vi "Double FFT Mesurament (Max Bin detection - Control - Init Wave&Window - Snapshot - DoubleFFT - Latency) test.vi"() -> ()   [LabVIEW 2014]
uses:
  <vilib>/Platform/TimedLoop/XDataNode/timing_clust.ctl
  <vilib>/Platform/TimedLoop/XDataNode/nitl_modes.ctl
  <vilib>/Platform/TimedLoop/XDataNode/wakeup.ctl
  <vilib>/rvi/Analysis/measure/FFT/simModelSupport/niFPGA FFT Streaming Sim Properties.ctl
  <vilib>/rvi/Analysis/measure/FFT/simModelSupport/niFPGA FFT Sim Stream Group Properties.ctl
  <vilib>/rvi/Analysis/measure/FFT/simModelSupport/niFPGA FFT Sim Types.ctl
  <vilib>/rvi/Analysis/measure/FFT/simModelSupport/niFpgaFFTSimArithmeticProperties.ctl
  <vilib>/rvi/Analysis/measure/FFT/simModelSupport/niFpgaFFTSimDfxp.ctl
  <vilib>/fxp/LVFixedPointQuantizationPolicyTypeDef.ctl
  <vilib>/rvi/Analysis/measure/FFT/XNode/niFpgaFFTButterflyDelays.ctl
  <vilib>/rvi/Emulation/niFpgaSctlEmulationGetInTimedLoop.vi
  <vilib>/rvi/Emulation/niFpgaEmulationReportErrorSimple.vi
  <vilib>/rvi/Emulation/niFpgaGetClockAttributes.vi
  <vilib>/rvi/Emulation/niFpgaCriticalErrorInLSC.vi
  <vilib>/rvi/Emulation/niFpgaEmulationIsFPGAContextNoSignature.vi
  <vilib>/rvi/DataTransferAndStorage/Container/Common/niFpgaContainerGetUniqueNameForEmu.vi
  <vilib>/rvi/Memory/Memory_Emulation/niFpgaMemoryEmulationCacheClearOnFirstRun.vi
  <vilib>/rvi/Memory/Memory_Emulation/nirvimemoryEmulationManagerCache_MakeExclusive.vi
  <vilib>/rvi/Memory/Memory_Emulation/niFpgaMemoryEmulationValidateCache.vi
  <vilib>/rvi/Memory/Memory_Emulation/nirvimemoryEmulationManagerCache_InsertValue.vi
  <vilib>/Utility/error.llb/Clear Errors.vi
  <vilib>/rvi/Memory/Memory_Emulation/nirvimemoryEmulationManagerCache_ReleaseExclusive.vi
  <vilib>/rvi/Memory/Memory_Emulation/nirvimemoryEmulationManagerCache_GetValue.vi
  <vilib>/rvi/Memory/Memory_Emulation/nirvimemoryEmulationManagerCache_SetValue.vi
  <vilib>/rvi/Emulation/niFpgaProcessEmulError.vi
  <vilib>/rvi/errors/niFpgaSetErrorForExecOnDevCompSimple.vi
  <vilib>/rvi/eio/common/nirviEmuReportErrorAndStop.vi
  <vilib>/rvi/FIFO/Fifo_Resource/nirvififoEmulationSetSize.vi
  <vilib>/rvi/FIFO/Fifo_Resource/nirviFifoEmulationQueueMgr.vi
  <instcachedir>/0/nirviFifoEmulationQueueMgr_E5CAEC123FF24DC58D834DCA3CDAA9B5.lvgen/nirviFifoEmulationQueueMgr_E5CAEC123FF24DC58D834DCA3CDAA9B5_012.vi
  <vilib>/rvi/FIFO/Fifo_Resource/nirvififoEmulationCreateLock.vi
  <vilib>/rvi/FIFO/Fifo_Resource/nirvififoEmulationObtainLock.vi
  <vilib>/rvi/FIFO/Fifo_Resource/nirvififoEmulationReleaseLock.vi
  <vilib>/rvi/occurrence/nirviWaitOnOccurrenceBase.vi
  <vilib>/rvi/errors/nirviReportUnexpectedCaseInternalError.vi
  <vilib>/rvi/errors/nirviReportUnexpectedCaseInternalError (U32).vi
  <instcachedir>/0/nirviFifoEmulationQueueMgr_E5CAEC123FF24DC58D834DCA3CDAA9B5.lvgen/nirviFifoEmulationQueueMgr_E5CAEC123FF24DC58D834DCA3CDAA9B5_010.vi
  <vilib>/rvi/FIFO/Fifo_Resource/nirvififoEmulationDetermineInputValidOut.vi
  <vilib>/rvi/Memory/Memory_Emulation/nirvimemoryFastEmulation.vi
  <vilib>/rvi/Memory/Memory_Emulation/nirvimemoryEmulation.vi
  <vilib>/rvi/Analysis/measure/FFT/simModelSupport/niFpgaFFTSimModelStreamingCore.vi
  <vilib>/rvi/interface/RandomDataEmulation/niFpgaRandomDataHandleErrors.vi
  <vilib>/rvi/eio/common/nirviEmuTemplateMethod_errors.vi
  <vilib>/Platform/TimedLoop/XDataNode/XDataNode.xnode
  <vilib>/rvi/DataTransferAndStorage/Container/XNode/niFpgaContainer.xnode
  <vilib>/rvi/DataTransferAndStorage/Register/Emulation/niFpgaRegisterEmulation.vi
  <vilib>/rvi/FIFO/Fifo_Resource/nirvififoEmulationRead.vi
  <vilib>/rvi/FIFO/Fifo_Resource/nirvififoEmulationWrite.vi
  <vilib>/rvi/FIFO/Fifo_Resource/nirvififoEmulationGetNumberOfElementsToWrite.vi
  <vilib>/rvi/Analysis/measure/FFT/XNode/niFpgaFFT.xnode
  <vilib>/rvi/interface/RandomDataEmulation/nirviRandomDataFpgaReadWriteTemplate.vi
  <vilib>/eio/EIOMethodNode/EIOMethodNode.xnode
  <vilib>/Platform/TimedLoop/XDataNode/XDNodeRunTimeDep.lvlib
panel:
  in  "Latency points":u32
  in  "snapshot":bool
  in  "first bin":i32=4
  in  "last bin":i32=251
  in  "lower limit 2":u32=682
  in  "lower limit 1":u32=57
  in  "upper limit 2":u32=1193
  in  "upper limit 1":u32=568
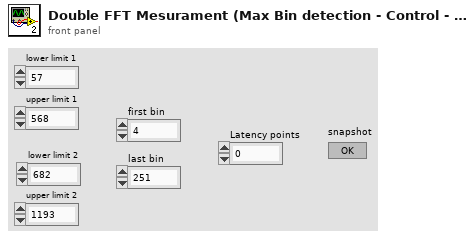
[diagram p1: front panel]
types:
  T1 = typedef "XDNodeRunTimeDep.lvlib/timing_clust.ctl" = cluster{"Expected End [f-1]":u64, "Actual End [f-1]":u64, "Finished Late? [f-1]":bool, "Expected End [i-1]":u64, "Actual End [i-1]":u64, "Finished Late? [i-1]":bool, "Expected Start [i]":u64, "Actual Start [i]":u64, "Expected Start [f]":u64, "Actual Start [f]":u64, "Source Name":string, "Structure Name":string, "Period":i64, "Deadline":i64, "Offset":i64, "Start":i64, "Priority":i32, "Timeout":i32, "Mode":T2, "Wakeup Reason":T3, "Error":errorcluster, "Source Type":string, "Secondary Source Type":string, "Global End Time":u64, "Global Start Time":u64, "Frame Duration":u64, "Iteration Duration":u64, "Assigned CPU":i32, "I/O Scan Engine Mode":u32}
  T2 = typedef "XDNodeRunTimeDep.lvlib/nitl_modes.ctl" = enum32{"No Change", "Process missed periods, maintain original phase", "Discard missed periods, maintain original phase", "Process missed periods, ignore original phase", "Discard missed periods, ignore original phase"}
  T3 = typedef "XDNodeRunTimeDep.lvlib/wakeup.ctl" = enum32{"Normal", "Aborted", "Asynchronous wakeup", "Timing source error", "Timed loop error", "Timeout"}
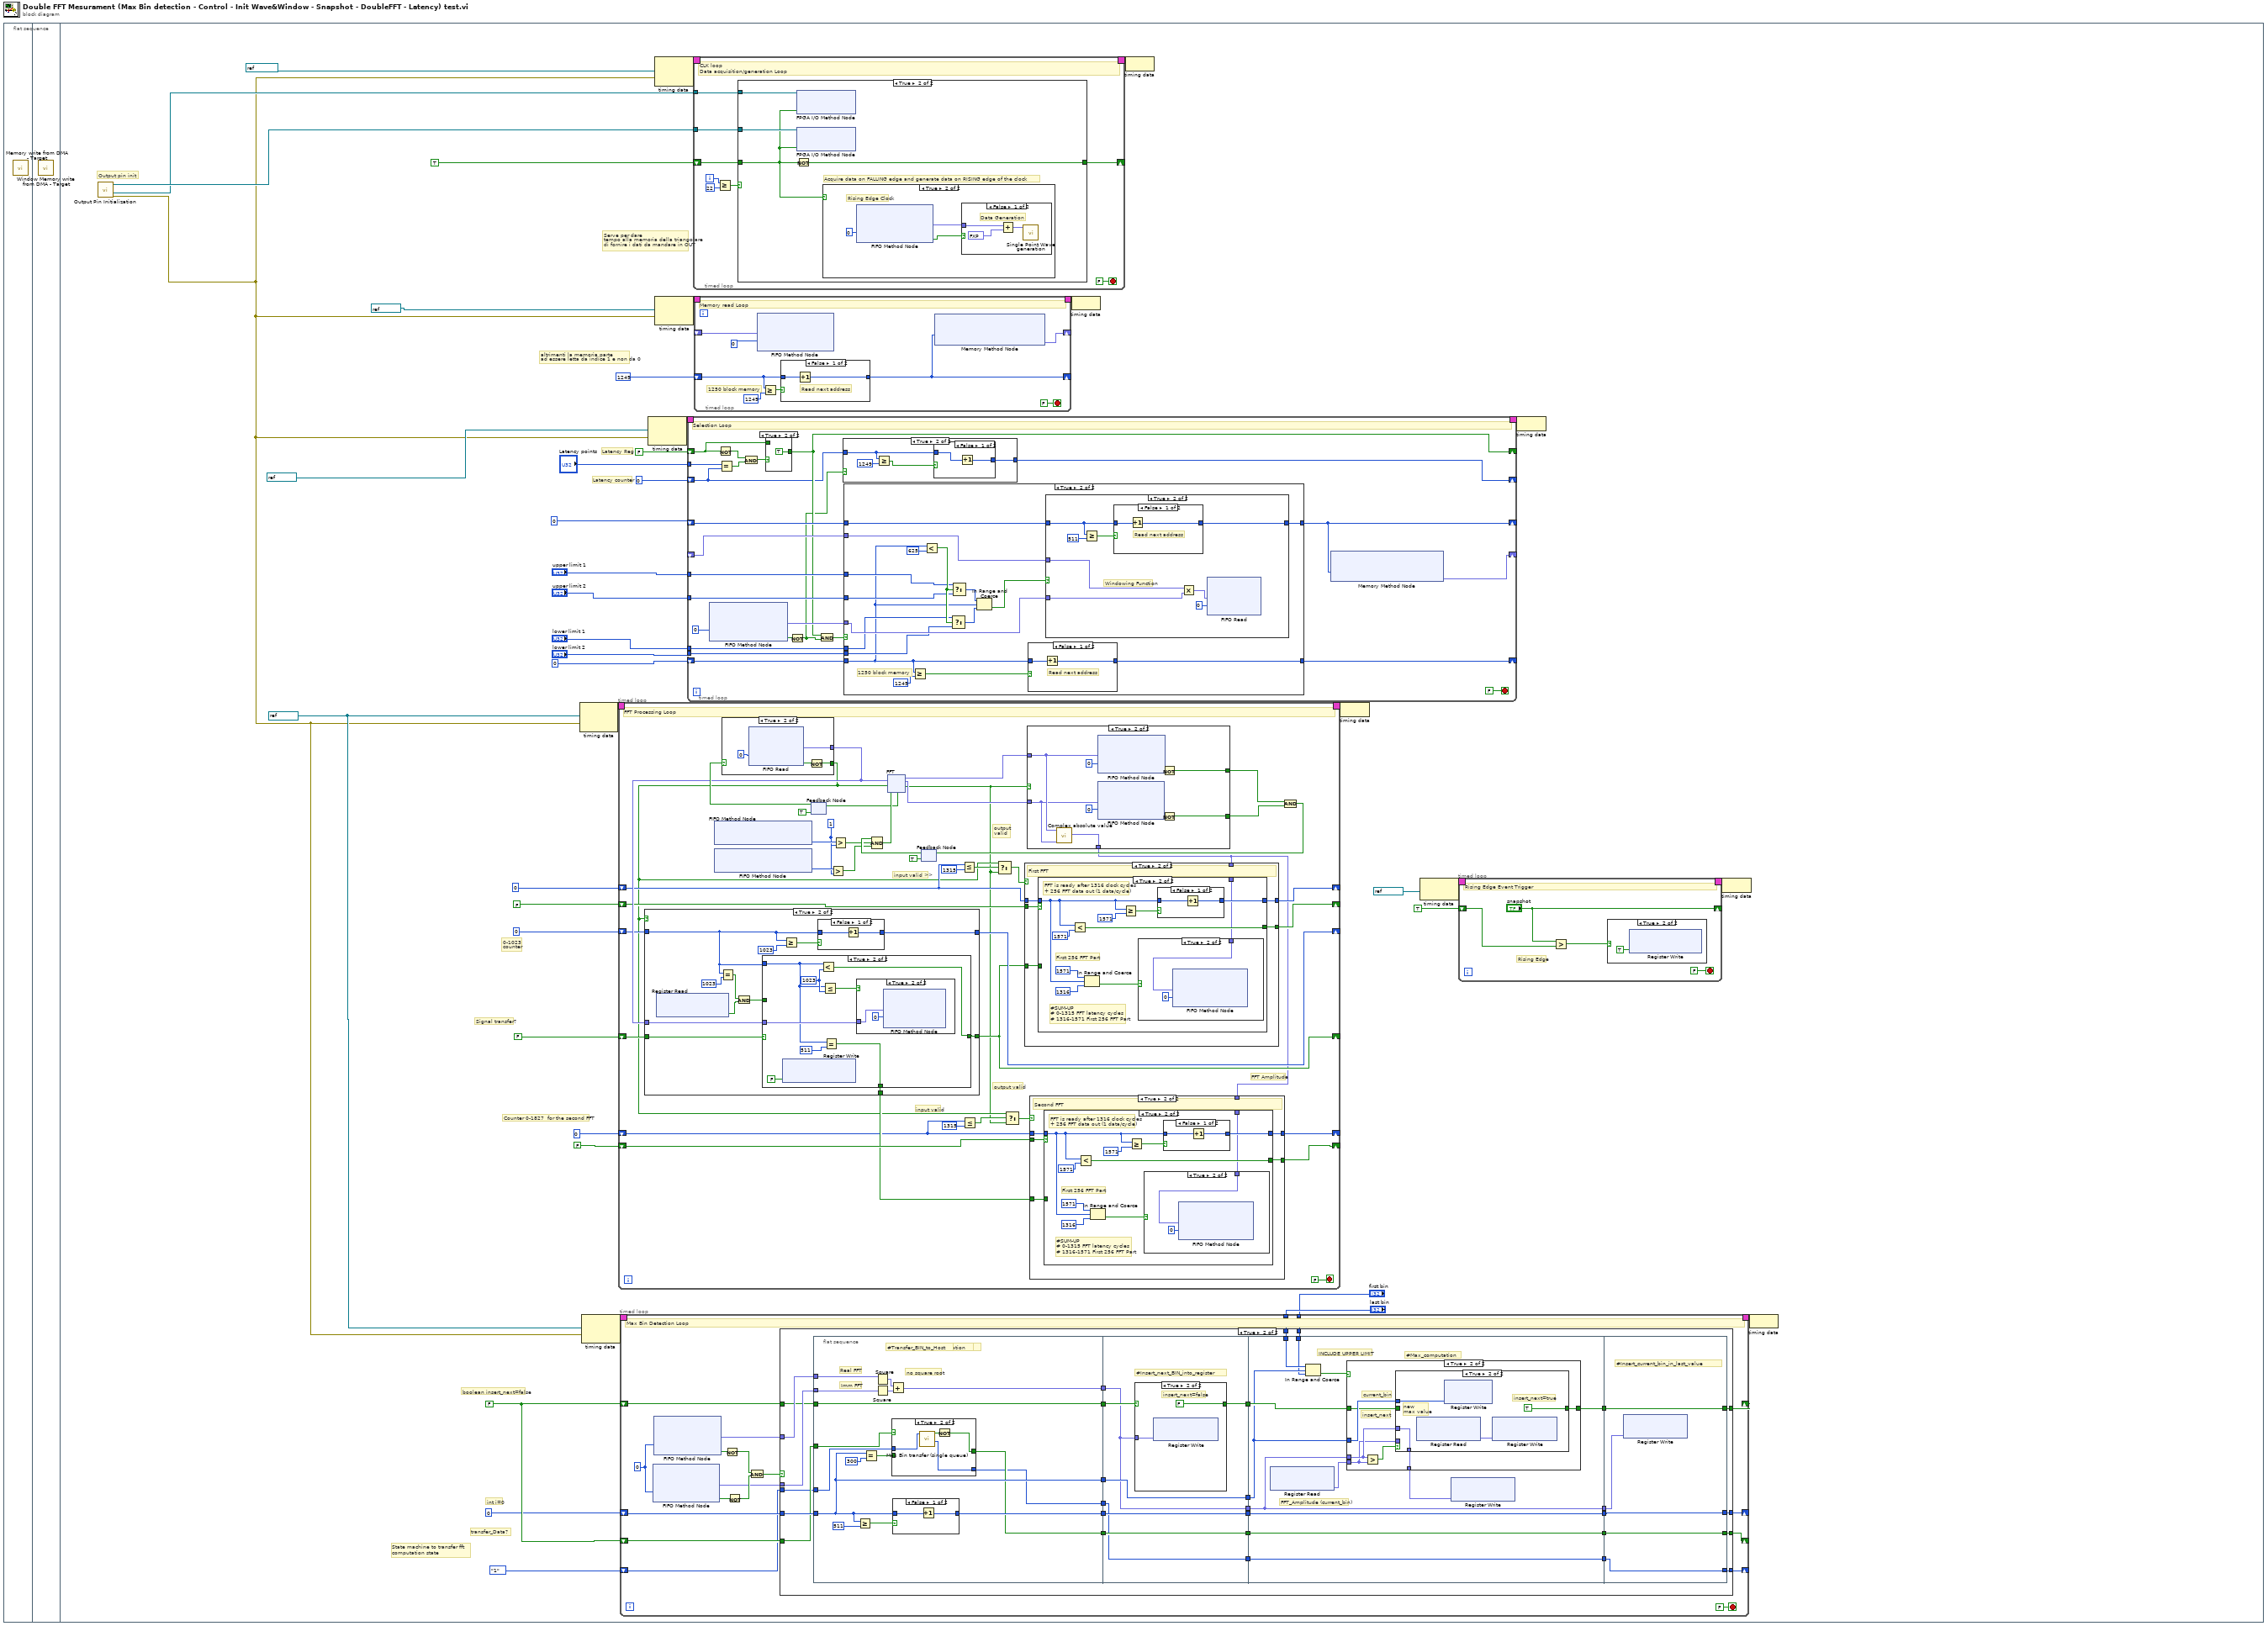
[diagram p0: block diagram]
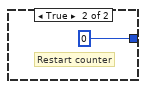
[diagram p5: hidden frame]
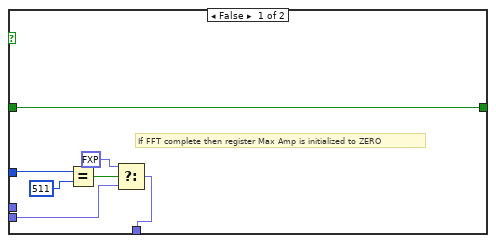
[diagram p7: hidden frame]
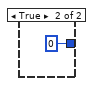
[diagram p10: hidden frame]
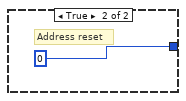
[diagram p14: hidden frame]
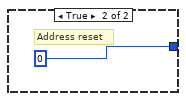
[diagram p15: hidden frame]
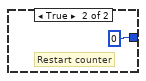
[diagram p19: hidden frame]
diagram:
  n1 = flat-sequence {
    frame #0 {
      n2 = call "Memory write from DMA - Target.vi"() -> ()  [unwired: 12 in]
    }
    frame #1 {
      n3 = call "Window Memory write from DMA - Target.vi"() -> ()  [unwired: 12 in]
    }
    frame #2 {
      w16 = FALSE
      w25 = refnum<k21> "50MHz" ("Source Name")
      # "altrimenti la memoria parte \nad essere letta da indice 1 e non da 0"
      # "Serve per dare\ntempo alla memoria della triangolare\ndi fornire i dati da mandare in OUT"
      # "Latency counter"
      # "Latency Reg"
      # "Counter 0-1827  for the second FFT"
      # "0-1023\ncounter"
      # "Signal transfer?"
      # "State machine to transfer fft\ncomputation state"
      # "transfer_Data?"
      # "int i=0"
      # "boolean insert_next=false"
      # "Output pin init"
      n4 = call "Output Pin Initialization.vi"() -> ("error out"=w24:errorcluster, "I/O Out Clock DAC (pin16)"=w28:refnum<k21>, "I/O Out Clock ADC (pin17)"=w29:refnum<k21>)  [unwired: 8 in]
      n5 = node-c288(w25, w24) -> (w39:T1)
      n6 = node-c288(w25, w24) -> (w35:T1)
      n7 = timed-loop {
        timing: w39 -> [_]
        timing-out: [_] -> w38
        shift-right: [w279] -> _
        shift-left: FALSE -> [w282]
        shift-right: [w283] -> _
        shift-left: i16 0 -> [w280]
        shift-right: [w278] -> _
        shift-left: FALSE -> [w277]
        shift-right: [w276] -> _
        shift-left: i16 0 -> [w274]
        shift-right: [w271] -> _
        shift-left: i16 0 -> [w264]
        shift-right: [w268] -> _
        shift-left: FALSE -> [w269]
        stop <- FALSE stop-if-true
        w286 = u32 1 ("y")
        # "output valid"
        # "input valid"
        # "FFT Amplitude"
        # "output\nvalid"
        # "input valid >>"
        # "FFT Processing Loop"
        n8 = xnode ("FIFO Method Node")() -> ("Number of Elements to Write"=w288:u32)  [unwired: 1 in, 1 out]
        n9 = xnode ("FIFO Method Node")() -> ("Number of Elements to Write"=w287:u32)  [unwired: 1 in, 1 out]
        n10 = feedback #1(TRUE ("ready for input")) -> (w300:bool)
        n11 = case shown="True" w300 {
          tunnel: [FALSE w422] -> w263
          tunnel: [fxp<+/-,12,12> 0.0 ("Element") w419] -> w281
          frame False {
            # "RMS is not ready for new input"
          }
          frame True {
            n12 = xnode ("FIFO Read")("Timeout"=0) -> ("Element"=w419:fxp<+/-,12,12>, "Timed Out?"=w421:bool)  [unwired: 1 in, 1 out]
            n13 = Not(x=w421) -> (.not. x?=w422:bool)
          }
        }
        n14 = case shown="True" w263 {
          tunnel: w280 -> [w353 w359]
          tunnel: [w353 w363] -> w283
          tunnel: w282 -> [w352 w357]
          tunnel: [w352 w358] -> w279
          tunnel: w281 -> [_ w356]
          tunnel: [FALSE w354] -> w267
          frame False {
          }
          frame True {
            n15 = xnode ("Register Read")() -> ("Data"=w355:bool)  [unwired: 1 in, 1 out]
            n16 = Equal?(x=w359, y=i16 1023) -> (x = y?=w362:bool)
            n17 = And(x=w362, y=w355) -> (x .and. y?=w360:bool)
            n18 = case shown="True" w357 {
              tunnel: w360 -> [w367 _]
              tunnel: w359 -> [_ w370]
              tunnel: [w367 w375] -> w358
              tunnel: w356 -> [_ w373]
              tunnel: [FALSE w368] -> w354
              frame False {
              }
              frame True {
                w372 = i16 1023 ("y")
                n19 = xnode ("Register Write")("Data"=FALSE) -> ()  [unwired: 1 in, 1 out]
                n20 = Less?(x=w370, y=w372) -> (x < y?=w375:bool)
                n21 = Less Or Equal?(x=w370, y=w372) -> (x <= y?=w374:bool)
                n22 = Equal?(x=w370, y=i16 511) -> (x = y?=w368:bool)
                n23 = case shown="True" w374 {
                  tunnel: w373 -> [_ w376]
                  frame False {
                  }
                  frame True {
                    n24 = xnode ("FIFO Method Node")("Element"=w376, "Timeout"=0) -> ()  [unwired: 1 in, 2 out]
                  }
                }
              }
            }
            n25 = Greater Or Equal?(x=w359, y=i16 1023) -> (x >= y?=w364:bool)
            n26 = case shown="False" w364 {
              tunnel: w359 -> [w379 _]
              tunnel: [w378 i16 0] -> w363
              frame False {
                n27 = Increment(x=w379) -> (x+1=w378:i16)
              }
              frame True {
                # "Restart counter"
              }
            }
          }
        }
        n28 = Greater?(x=w287, y=w286) -> (0:w284:bool)
        n29 = Greater?(x=w288, y=w286) -> (0:w285:bool)
        n30 = feedback #2(TRUE) -> (w296:bool)
        n31 = Compound Arithmetic op=AND(w296, w285, w284) -> (w295:bool)
        n32 = xnode "FFT"("real data in"=w281, "input valid"=w263, "ready for output"=w295) -> ("ready for input"=w294:bool, "real data out"=w293:fxp<+/-,22,22>, "imaginary data out"=w292:fxp<+/-,22,22>, "output valid"=w261:bool)  [unwired: 2 in, 1 out]
        n33 = feedback-in #1(w294) -> ()
        n34 = Less Or Equal?(x=w274, y=i16 1315) -> (x <= y?=w275:bool)
        n35 = Less Or Equal?(x=w264, y=i16 1315) -> (x <= y?=w265:bool)
        n36 = Select(t=w263, s=w275, f=w261) -> (s? t:f=w272:bool)
        n37 = Select(t=w263, s=w265, f=w261) -> (s? t:f=w262:bool)
        n38 = case shown="True" w261 {
          tunnel: w293 -> [_ w410]
          tunnel: w292 -> [_ w409]
          tunnel: [w407 w416] -> w291
          tunnel: [w407 w415] -> w290
          tunnel: [_ w408] -> w270
          frame False {
            w407 = TRUE
          }
          frame True {
            n39 = call "Complex absolute value.vi"("Im"=w409, "Re"=w410) -> ("Square Absolute Value"=w408:fxp<+,44,44>)  [unwired: 9 in]
            n40 = xnode ("FIFO Method Node")("Element"=w410, "Timeout"=0) -> ("Timed Out?"=w411:bool)  [unwired: 1 in, 1 out]
            n41 = xnode ("FIFO Method Node")("Element"=w409, "Timeout"=0) -> ("Timed Out?"=w412:bool)  [unwired: 1 in, 1 out]
            n42 = Not(x=w411) -> (.not. x?=w416:bool)
            n43 = Not(x=w412) -> (.not. x?=w415:bool)
          }
        }
        n44 = case shown="True" w272 {
          tunnel: w279 -> [_ w333]
          tunnel: [w326 w332] -> w278
          tunnel: w277 -> [w326 w331]
          tunnel: w274 -> [w327 w330]
          tunnel: [w327 w329] -> w276
          tunnel: w270 -> [_ w328]
          frame False {
          }
          frame True {
            # "First FFT"
            n45 = case shown="True" w331 {
              tunnel: w333 -> [w335 _]
              tunnel: [w335 w345] -> w332
              tunnel: w330 -> [w334 w338]
              tunnel: [w334 w341] -> w329
              tunnel: w328 -> [_ w336]
              frame False {
              }
              frame True {
                # "First 256 FFT Part"
                # "#SUM-UP\n# 0-1315 FFT latency cycles\n# 1316-1571 First 256 FFT Part"
                # "FFT is ready after 1316 clock cycles\n+ 256 FFT data out (1 data/cycle)"
                n46 = Less?(x=w338, y=i16 1571) -> (x < y?=w345:bool)
                n47 = In Range and Coerce(upper limit=i16 1571, x=w338, lower limit=i16 1316 ("y")) -> (In Range?=w337:bool)  [unwired: 1 out]
                n48 = Greater Or Equal?(x=w338, y=i16 1571) -> (x >= y?=w342:bool)
                n49 = case shown="True" w337 {
                  tunnel: w336 -> [_ w347]
                  frame False {
                  }
                  frame True {
                    n50 = xnode ("FIFO Method Node")("Element"=w347, "Timeout"=0) -> ()  [unwired: 1 in, 2 out]
                  }
                }
                n51 = case shown="False" w342 {
                  tunnel: w338 -> [w349 _]
                  tunnel: [w348 i16 0] -> w341
                  frame False {
                    n52 = Increment(x=w349) -> (x+1=w348:i16)
                  }
                  frame True {
                    # "Restart counter"
                  }
                }
              }
            }
          }
        }
        n53 = case shown="True" w262 {
          tunnel: w267 -> [_ w308]
          tunnel: [w301 w307] -> w268
          tunnel: w269 -> [w301 w306]
          tunnel: w264 -> [w302 w305]
          tunnel: [w302 w304] -> w271
          tunnel: w270 -> [_ w303]
          frame False {
          }
          frame True {
            # "Second FFT"
            n54 = case shown="True" w306 {
              tunnel: w308 -> [w310 _]
              tunnel: [w310 w320] -> w307
              tunnel: w305 -> [w309 w313]
              tunnel: [w309 w316] -> w304
              tunnel: w303 -> [_ w311]
              frame False {
              }
              frame True {
                # "First 256 FFT Part"
                # "#SUM-UP\n# 0-1315 FFT latency cycles\n# 1316-1571 First 256 FFT Part"
                # "FFT is ready after 1316 clock cycles\n+ 256 FFT data out (1 data/cycle)"
                n55 = Less?(x=w313, y=i16 1571) -> (x < y?=w320:bool)
                n56 = In Range and Coerce(upper limit=i16 1571, x=w313, lower limit=i16 1316 ("y")) -> (In Range?=w312:bool)  [unwired: 1 out]
                n57 = Greater Or Equal?(x=w313, y=i16 1571) -> (x >= y?=w317:bool)
                n58 = case shown="True" w312 {
                  tunnel: w311 -> [_ w322]
                  frame False {
                  }
                  frame True {
                    n59 = xnode ("FIFO Method Node")("Element"=w322, "Timeout"=0) -> ()  [unwired: 1 in, 2 out]
                  }
                }
                n60 = case shown="False" w317 {
                  tunnel: w313 -> [w324 _]
                  tunnel: [w323 i16 0] -> w316
                  frame False {
                    n61 = Increment(x=w324) -> (x+1=w323:i16)
                  }
                  frame True {
                    # "Restart counter"
                  }
                }
              }
            }
          }
        }
        n62 = Compound Arithmetic op=AND(w291, w290) -> (w289:bool)
        n63 = feedback-in #2(w289) -> ()
      }
      n64 = timed-loop {
        shift-right: [w65] -> _
        shift-left: 0 ("Timeout") -> [w66]
        shift-right: [w63] -> _
        shift-left: w16 -> [w64]
        timing: w35 -> [_]
        timing-out: [_] -> w34
        tunnel: "last bin" -> [w61]
        tunnel: "first bin" -> [w60]
        shift-right: [w57] -> _
        shift-left: w16 -> [w58]
        shift-right: [w55] -> _
        shift-left: enum16{"1", "2", "3", "4"}."1" ("Enum") -> [w56]
        stop <- FALSE stop-if-true
        w59 = 0 ("Timeout")
        # "Max Bin Detection Loop"
        n65 = xnode ("FIFO Method Node")("Timeout"=w59) -> ("Element"=w67:fxp<+/-,22,22>, "Timed Out?"=w72:bool)  [unwired: 1 in, 1 out]
        n66 = xnode ("FIFO Method Node")("Timeout"=w59) -> ("Element"=w68:fxp<+/-,22,22>, "Timed Out?"=w73:bool)  [unwired: 1 in, 1 out]
        n67 = Not(x=w73) -> (.not. x?=w71:bool)
        n68 = Not(x=w72) -> (.not. x?=w70:bool)
        n69 = And(x=w71, y=w70) -> (x .and. y?=w69:bool)
        n70 = case shown="True" w69 {
          tunnel: w68 -> [_ w106]
          tunnel: w67 -> [_ w105]
          tunnel: w66 -> [w77 w103]
          tunnel: [w77 w90] -> w65
          tunnel: w64 -> [w76 w97]
          tunnel: [w76 w92] -> w63
          tunnel: w61 -> [_ w89]
          tunnel: w60 -> [_ w88]
          tunnel: w58 -> [w75 w87]
          tunnel: [w75 w86] -> w57
          tunnel: w56 -> [w74 w82]
          tunnel: [w74 w78] -> w55
          frame False {
            # "Data are NOT ready in Target Real FFT and Target Imm FFT FIFOs"
          }
          frame True {
            n71 = flat-sequence {
              tunnel: w106 -> [w119]
              tunnel: w105 -> [w120]
              tunnel: [w113] -> w104
              tunnel: w103 -> [w112]
              tunnel: [w118] -> w102
              tunnel: [w112] -> w99
              tunnel: [w115] -> w98
              tunnel: w97 -> [w115]
              tunnel: w87 -> [w111]
              tunnel: [w109] -> w85
              tunnel: w82 -> [w108]
              tunnel: [w107] -> w79
              tunnel: w104 -> [w135]
              tunnel: w102 -> [w138]
              tunnel: [w138] -> w101
              tunnel: w99 -> [w136]
              tunnel: w98 -> [w137]
              tunnel: [w136] -> w96
              tunnel: [w135] -> w95
              tunnel: [w134] -> w94
              tunnel: w85 -> [w133]
              tunnel: [w133] -> w84
              tunnel: [w132] -> w80
              tunnel: w79 -> [w132]
              tunnel: w101 -> [w153]
              tunnel: [w153] -> w100
              tunnel: w96 -> [w148]
              tunnel: w95 -> [w150]
              tunnel: w94 -> [w151]
              tunnel: [w150] -> w93
              tunnel: [w149] -> w91
              tunnel: w89 -> [w145]
              tunnel: w88 -> [w144]
              tunnel: w84 -> [w143]
              tunnel: [w143] -> w83
              tunnel: [w142] -> w81
              tunnel: w80 -> [w142]
              tunnel: w100 -> [w176]
              tunnel: w93 -> [w178]
              tunnel: w91 -> [w177]
              tunnel: [w177] -> w92
              tunnel: [w176] -> w90
              tunnel: [w175] -> w86
              tunnel: w83 -> [w175]
              tunnel: w81 -> [w174]
              tunnel: [w174] -> w78
              frame #0 {
                # "no square root"
                # "#Transfer_BIN_to_Host"
                # "#Iteration_Counter_Computation"
                # "#FFT_Amplitude_Computation"
                # "Imm FFT"
                # "Real FFT"
                n72 = Greater Or Equal?(x=w112, y=511) -> (x >= y?=w116:bool)
                n73 = Equal?(x=w112, y=300) -> (x = y?=w110:bool)
                n74 = Square(x=w119) -> (x^2=w122:fxp<+,43,43>)
                n75 = Square(x=w120) -> (x^2=w121:fxp<+,43,43>)
                n76 = Add(x=w122, y=w121) -> (x+y=w113:fxp<+,44,44>)
                n77 = case shown="True" w111 {
                  tunnel: w110 -> [w124 _]
                  tunnel: [w124 w127] -> w109
                  tunnel: w108 -> [w123 w126]
                  tunnel: [w123 w125] -> w107
                  frame False {
                    # "FFT Comp is NOT finished"
                  }
                  frame True {
                    n78 = call "Max Bin transfer (single queue).vi"("Enum"=w126) -> ("Next state"=w125:enum16{"1", "2", "3", "4"}, "END?"=w128:bool)  [unwired: 9 in]
                    n79 = Not(x=w128) -> (.not. x?=w127:bool)
                  }
                }
                n80 = case shown="False" w116 {
                  tunnel: w112 -> [w129 _]
                  tunnel: [w130 0 ("Timeout")] -> w118
                  frame False {
                    n81 = Increment(x=w129) -> (x+1=w130:i32)
                  }
                  frame True {
                    # "Restart counter"
                  }
                }
              }
              frame #1 {
                # "#Insert_next_BIN_into_register"
                n82 = case shown="True" w137 {
                  selector: w137 -> [w139 _]
                  tunnel: [w139 FALSE] -> w134
                  tunnel: w135 -> [_ w140]
                  frame False {
                  }
                  frame True {
                    # "insert_next=false"
                    n83 = xnode ("Register Write")("Data"=w140) -> ()  [unwired: 1 in, 1 out]
                  }
                }
              }
              frame #2 {
                # "INCLUDE UPPER LIMIT"
                # "FFT_Amplitude (current_bin)"
                # "#Max_computation"
                n84 = xnode ("Register Read")() -> ("Data"=w147:fxp<+,44,44>)  [unwired: 1 in, 1 out]
                n85 = In Range and Coerce(upper limit=w145, x=w148, lower limit=w144) -> (In Range?=w152:bool)  [unwired: 1 out]
                n86 = case shown="True" w152 {
                  tunnel: w150 -> [_ w166]
                  tunnel: w148 -> [w158 w165]
                  tunnel: w151 -> [w160 w164]
                  tunnel: [w160 w163] -> w149
                  tunnel: w147 -> [w156 w161]
                  tunnel: [w154 w162] -> w146
                  frame False {
                    # "If FFT complete then register Max Amp is initialized to ZERO"
                    n87 = Equal?(x=w158, y=511) -> (x = y?=w159:bool)
                    n88 = Select(t=fxp<+,44,44> 0.0, s=w159, f=w156) -> (s? t:f=w154:fxp<+,44,44>)
                  }
                  frame True {
                    # "insert_next"
                    # "current_bin"
                    n89 = Greater?(x=w166, y=w161) -> (0:w167:bool)
                    n90 = case shown="True" w167 {
                      tunnel: w166 -> [_ w170]
                      tunnel: w165 -> [_ w173]
                      tunnel: w164 -> [w169 _]
                      tunnel: [w169 TRUE] -> w163
                      tunnel: [w168 w170] -> w162
                      tunnel: w161 -> [w168 _]
                      frame False {
                        # "Old value is re-written"
                      }
                      frame True {
                        # "new\nmax value"
                        # "insert_next=true"
                        n91 = xnode ("Register Read")() -> ("Data"=w171:fxp<+,44,44>)  [unwired: 1 in, 1 out]
                        n92 = xnode ("Register Write")("Data"=w173) -> ()  [unwired: 1 in, 1 out]
                        n93 = xnode ("Register Write")("Data"=w171) -> ()  [unwired: 1 in, 1 out]
                      }
                    }
                  }
                }
                n94 = xnode ("Register Write")("Data"=w146) -> ()  [unwired: 1 in, 1 out]
              }
              frame #3 {
                # "#Insert_current_bin_in_last_value"
                n95 = xnode ("Register Write")("Data"=w178) -> ()  [unwired: 1 in, 1 out]
              }
            }
          }
        }
      }
      n96 = node-c288(refnum<k21> "50MHz" ("Source Name"), w24) -> (w37:T1)
      n97 = node-c288(refnum<k21> "100MHz" ("Source Name"), w24) -> (w43:T1)
      n98 = node-c288(refnum<k21> "50MHz" ("Source Name"), w24) -> (w41:T1)
      n99 = timed-loop {
        timing: w37 -> [_]
        timing-out: [_] -> w36
        shift-right: [w208] -> _
        shift-left: u32 0 -> [w195]
        tunnel: "upper limit 1" -> [w204]
        tunnel: "upper limit 2" -> [w203]
        tunnel: "lower limit 1" -> [w202]
        tunnel: "lower limit 2" -> [w201]
        shift-right: [w197] -> _
        shift-left: u32 0 -> [w200]
        shift-right: [w198] -> _
        shift-left: _ -> [w199]
        shift-right: [w189] -> _
        shift-left: FALSE -> [w190]
        tunnel: "Latency points" -> [w194]
        shift-right: [w187] -> _
        shift-left: u32 0 -> [w186]
        stop <- FALSE stop-if-true
        # "Selection Loop"
        n100 = xnode ("FIFO Method Node")("Timeout"=0) -> ("Element"=w206:fxp<+/-,12,12>, "Timed Out?"=w207:bool)  [unwired: 1 in, 1 out]
        n101 = Not(x=w190) -> (.not. x?=w193:bool)
        n102 = Equal?(x=w194, y=w186) -> (x = y?=w192:bool)
        n103 = And(x=w193, y=w192) -> (x .and. y?=w191:bool)
        n104 = case shown="True" w191 {
          tunnel: [w218 TRUE] -> w189
          tunnel: w190 -> [w218 _]
          frame False {
          }
          frame True {
          }
        }
        n105 = Not(x=w207) -> (.not. x?=w188:bool)
        n106 = And(x=w189, y=w188) -> (x .and. y?=w196:bool)
        n107 = case shown="True" w188 {
          tunnel: w186 -> [w210 w213]
          tunnel: [w210 w211] -> w187
          frame False {
          }
          frame True {
            n108 = Greater Or Equal?(x=w213, y=u32 1249) -> (x >= y?=w212:bool)
            n109 = case shown="False" w212 {
              tunnel: w213 -> [w216 _]
              tunnel: [w215 u32 0] -> w211
              frame False {
                n110 = Increment(x=w216) -> (x+1=w215:u32)
              }
              frame True {
              }
            }
          }
        }
        n111 = case shown="True" w196 {
          tunnel: [w221 w236] -> w208
          tunnel: w195 -> [w221 w223]
          tunnel: w206 -> [_ w231]
          tunnel: w204 -> [_ w230]
          tunnel: w203 -> [_ w229]
          tunnel: w202 -> [_ w228]
          tunnel: w201 -> [_ w227]
          tunnel: w200 -> [w220 w224]
          tunnel: [w220 w226] -> w197
          tunnel: w199 -> [_ w225]
          frame False {
          }
          frame True {
            # "1250 block memory"
            n112 = Greater Or Equal?(x=w223, y=u32 1249) -> (x >= y?=w237:bool)
            n113 = Less?(x=w223, y=u32 625) -> (x < y?=w232:bool)
            n114 = Select(t=w228, s=w232, f=w227) -> (s? t:f=w234:u32)
            n115 = Select(t=w230, s=w232, f=w229) -> (s? t:f=w235:u32)
            n116 = In Range and Coerce(upper limit=w235, x=w223, lower limit=w234) -> (In Range?=w222:bool)  [unwired: 1 out]
            n117 = case shown="False" w237 {
              tunnel: w223 -> [w252 _]
              tunnel: [w251 u32 0] -> w236
              frame False {
                # "Read next address"
                n118 = Increment(x=w252) -> (x+1=w251:u32)
              }
              frame True {
                # "Address reset"
              }
            }
            n119 = case shown="True" w222 {
              tunnel: w231 -> [_ w240]
              tunnel: w224 -> [w239 w245]
              tunnel: [w239 w247] -> w226
              tunnel: w225 -> [_ w243]
              frame False {
              }
              frame True {
                # "Windowing Function"
                n120 = Greater Or Equal?(x=w245, y=u32 511) -> (x >= y?=w246:bool)
                n121 = case shown="False" w246 {
                  tunnel: w245 -> [w249 _]
                  tunnel: [w248 u32 0] -> w247
                  frame False {
                    # "Read next address"
                    n122 = Increment(x=w249) -> (x+1=w248:u32)
                  }
                  frame True {
                    # "Address reset"
                  }
                }
                n123 = Multiply(x=w243, y=w240) -> (x*y=w241:fxp<+/-,12,12>)
                n124 = xnode ("FIFO Read")("Element"=w241, "Timeout"=0) -> ()  [unwired: 1 in, 2 out]
              }
            }
          }
        }
        n125 = xnode ("Memory Method Node")("Address"=w197) -> ("Data"=w198:fxp<+,8,1>)  [unwired: 1 in, 1 out]
      }
      n126 = timed-loop {
        timing: w43 -> [_]
        timing-out: [_] -> w42
        shift-right: [w453] -> _
        shift-left: TRUE -> [w451]
        tunnel: w28 -> [w455]
        tunnel: w29 -> [w452]
        i -> [w449]
        stop <- FALSE stop-if-true
        # "CLK loop\nData acquisition/generation Loop"
        n127 = Greater Or Equal?(x=w449, y=22) -> (x >= y?=w448:bool)
        n128 = case shown="True" w448 {
          tunnel: w455 -> [_ w460]
          tunnel: [w456 w459] -> w453
          tunnel: w452 -> [_ w458]
          tunnel: w451 -> [w456 w457]
          frame False {
          }
          frame True {
            # "Acquire data on FALLING edge and generate data on RISING edge of the clock"
            n129 = Not(x=w457) -> (.not. x?=w459:bool)
            n130 = xnode "FPGA I/O Method Node"("FPGA I/O In"=w460, "Data"=w457) -> ()  [unwired: 1 out]
            n131 = xnode "FPGA I/O Method Node"("FPGA I/O In"=w458, "Data"=w457) -> ()  [unwired: 1 out]
            n132 = case shown="True" w457 {
              frame False {
                # "Falling Edge Clock"
                n133 = call "Single Acquisition.vi"() -> ("Out"=w462:fxp<+/-,12,12>)  [unwired: 10 in, 1 out]
                n134 = xnode ("FIFO Method Node")("Element"=w462, "Timeout"=0) -> ()  [unwired: 1 in, 2 out]
              }
              frame True {
                # "Rising Edge Clock"
                n135 = xnode ("FIFO Method Node")("Timeout"=0) -> ("Element"=w463:fxp<+/-,12,12>, "Timed Out?"=w464:bool)  [unwired: 1 in, 1 out]
                n136 = case shown="False" w464 {
                  tunnel: w463 -> [w468 _]
                  frame False {
                    # "Data Generation"
                    n137 = Add(x=w468, y=fxp<+,12,12> 2048.0) -> (x+y=w466:fxp<+/-,14,14>)
                    n138 = call "Single Point Wave generation.vi"("Data To Write"=w466) -> ()  [unwired: 10 in, 1 out]
                  }
                  frame True {
                    # "FPGA memory slow"
                  }
                }
              }
            }
          }
        }
      }
      n139 = timed-loop {
        timing: w41 -> [_]
        timing-out: [_] -> w40
        shift-right: [w430] -> _
        shift-left: u32 1249 -> [w434]
        shift-right: [w432] -> _
        shift-left: _ -> [w431]
        stop <- FALSE stop-if-true
        # "1250 block memory"
        # "Memory read Loop"
        n140 = xnode ("FIFO Method Node")("Element"=w431, "Timeout"=0) -> ()  [unwired: 1 in, 2 out]
        n141 = Greater Or Equal?(x=w434, y=u32 1249) -> (x >= y?=w436:bool)
        n142 = case shown="False" w436 {
          tunnel: w434 -> [w439 _]
          tunnel: [w438 u32 0] -> w430
          frame False {
            # "Read next address"
            n143 = Increment(x=w439) -> (x+1=w438:u32)
          }
          frame True {
            # "Address reset"
          }
        }
        n144 = xnode ("Memory Method Node")("Address"=w430) -> ("Data"=w432:fxp<+/-,12,12>)  [unwired: 1 in, 1 out]
      }
      n145 = node-c288(w40) -> ()
      n146 = node-c288(w42) -> ()
      n147 = node-c288(w38) -> ()
      n148 = node-c288(refnum<k21> "50MHz" ("Source Name")) -> (w9:T1)
      n149 = timed-loop {
        timing: w9 -> [_]
        timing-out: [_] -> w8
        shift-right: ["snapshot"] -> _
        shift-left: TRUE ("snapshot") -> [w46]
        stop <- FALSE stop-if-true
        # "Rising Edge"
        # "Rising Edge Event Trigger"
        n150 = Greater?(x="snapshot", y=w46) -> (0:w44:bool)
        n151 = case shown="True" w44 {
          frame False {
          }
          frame True {
            n152 = xnode ("Register Write")("Data"=TRUE) -> ()  [unwired: 1 in, 1 out]
          }
        }
      }
      n153 = node-c288(w36) -> ()
      n154 = node-c288(w8) -> ()
      n155 = node-c288(w34) -> ()
    }
  }
